vi "PH_Beckhoff_Common.create Beckhoff BB Tagnames.vi"(0 "#":i32, 1 "Instance Name":string) -> (2 "Input Tags":string[](array[string]), 3 "move-in-Tags":string[](array[string]), 4 "move-Tags":string[](array[string]))   [LabVIEW 2014, in "PH_Beckhoff_Common.lvlib"]
doc: "This VI creates Black Box Tagnames:\n\n\"Input Tags\": Array of \n<Instancename>_BB_1_remote_controlled\n<Instancename>_BB_1_out\n<Instancename>_BB_1_in\n...\n<Instancename>_BB_#_remote_controlled\n<Instancename>_BB_#_out\n<Instancename>_BB_#_in\n\n\"move-in-Tags: Array of\n<Instancename>_BB_1_move_in\n...\n<Instancename>_BB_#__move_in\n\n\"move-Tags\": Array of\n<Instancename>_BB_1_move\n...\n<Instancename>_BB_#_move"
uses:
  PH_Beckhoff_Common.lvlib
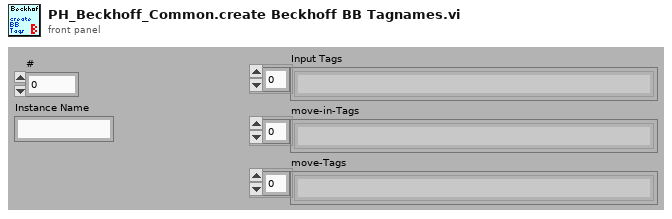
[diagram p1: front panel]
types:
  T1 = typedef "PH_Beckhoff_Common.lvlib/PH_Beckhoff_Common.BB Tagnames.ctl" = cluster{"Sensor Remote controlled":string, "Sensor Out":string, "Sensor In":string, "Actor Direction In":string, "Actor Move":string, "Sensor Power ok":string, "Instance":string}
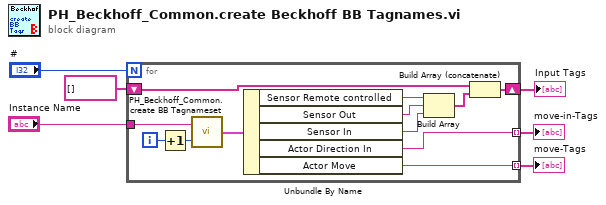
[diagram p0: block diagram]
diagram:
  n1 = for {
    N: "#" -> [_]
    tunnel: [w8] -> w4 mode=indexing
    tunnel: [w7] -> w3 mode=indexing
    tunnel: "Instance Name" -> [w16]
    shift-right: [w15] -> w1
    shift-left: string[] [] -> [w14]
    i -> [w18]
    n2 = Increment(x=w18) -> (x+1=w17:i32)
    n3 = call "PH_Beckhoff_Common.create BB Tagnameset.vi"("#"=w17, "Instance Name"=w16) -> ("output cluster"=w13:T1)
    n4 = Unbundle By Name(w13) -> ("Sensor Remote controlled"=w12:string, "Sensor Out"=w11:string, "Sensor In"=w10:string, "Actor Direction In"=w8:string, "Actor Move"=w7:string)
    n5 = Build Array(w12, w11, w10) -> (w9:string[])
    n6 = Build Array (concatenate)(w14, w9) -> (w15:string[])
  }
  "move-in-Tags" <- w4
  "move-Tags" <- w3
  "Input Tags" <- w1
